vi "Write Recipe.vi"(8 "error in (no error)":errorcluster, 11 "Masterv2 in":refnum<class "Masterv2.lvclass">) -> (0 "error out":errorcluster, 3 "Masterv2 out":refnum<class "Masterv2.lvclass">)   [LabVIEW 2014, in "Main Libraryv2.lvlib" / "Masterv2.lvclass"]
uses:
  Master/Masterv2.lvclass
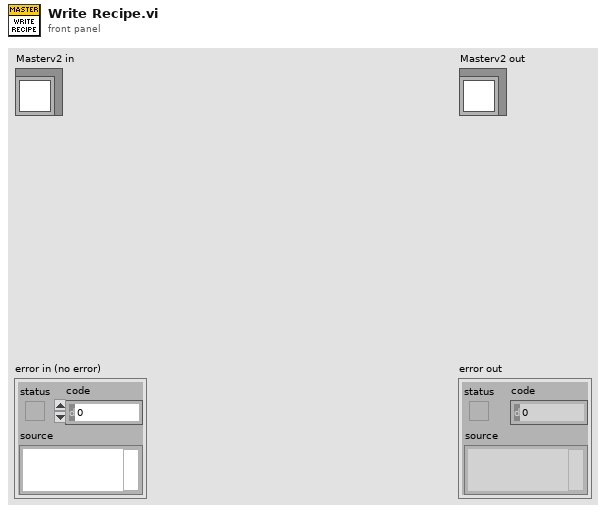
[diagram p1: front panel]
types:
  T1 = cluster{"Speed":string, "Temperature SP":string, "Time Limit":string, "Direction":string}[]
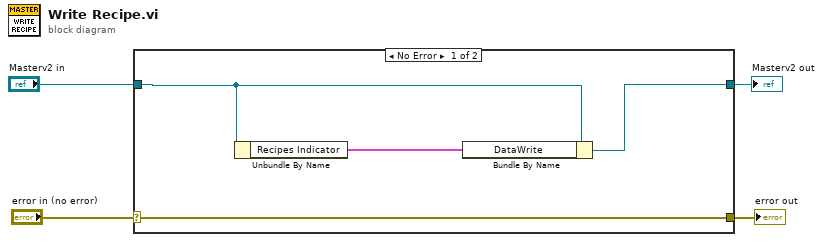
[diagram p0: block diagram]
diagram:
  n1 = case shown="No Error" "error in (no error)" {
    selector: "error in (no error)" -> [w8 w10]
    tunnel: [w8 w10] -> w3
    tunnel: [w5 w9] -> w1
    tunnel: "Masterv2 in" -> [w6 w9]
    frame No Error {
      n2 = Unbundle By Name(w6) -> ("Recipes Indicator"=w7:T1)
      n3 = Bundle By Name(cluster=w6, "DataWrite"=w7) -> (w5:refnum<class "Masterv2.lvclass">)
    }
    frame Error {
    }
  }
  "error out" <- w3
  "Masterv2 out" <- w1
